vi "PCO_SetADCOperation.vi"(8 "error in (no error)":errorcluster {"code" format="%x"}, 10 "wADCOperation":u16(ring) items=["", "single ADC", "dual ADC"], 11 "ph":u64) -> (0 "error out":errorcluster {"code" format="%x"}, 2 "ErrorMessage":i32 format="%x", 3 "ph out":u64)   [LabVIEW 2019, in "SDK.lvlib" / "ImageSensor.lvlib"]
doc: "<b>Description:</b>\nThis function does set the ADC (analog-digital-converter) operating mode. Possible values are given through the parameter wNumADCsDESC of the PCO_Description structure. If sensor data is read out using single ADC operation linearity of image data is enhanced, using dual ADC operation readout is faster and allows higher frame rates. If dual ADC operating mode is set, horizontal ROI must be adapted to symmetrical values.\n\n<b>Supported camera type:</b>\npco.1600, pco.2000, pco.4000\n\n<b>Descriptor dependency:</b>\nwNumADCsDESC"
uses:
  ImageSensor.lvlib
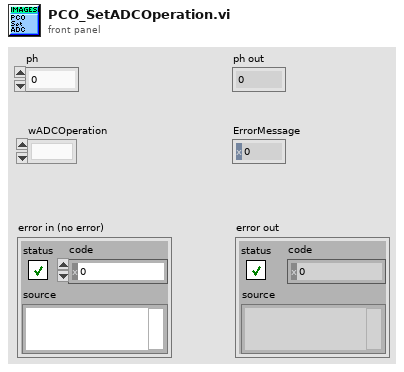
[diagram p1: front panel]
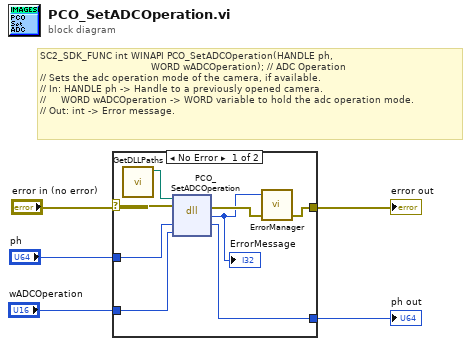
[diagram p0: block diagram]
diagram:
  # "SC2_SDK_FUNC int WINAPI PCO_SetADCOperation(HANDLE ph,\n                                     WORD wADCOperation); // ADC Operation\n// Sets the adc operation mode of the camera, if available.\n// In: HANDLE ph -> Handle to a previously opened camera.\n//     WORD wADCOperation -> WORD variable to hold the adc operation mode.\n// Out: int -> Error message."
  n1 = case shown="No Error" "error in (no error)" {
    selector: "error in (no error)" -> [w10 w15]
    tunnel: "ph" -> [w13 w14]
    tunnel: [w12 w14] -> w4
    tunnel: "wADCOperation" -> [w11 _]
    tunnel: [w8 w15] -> w2
    frame No Error {
      n2 = call "GetDLLPaths.vi"() -> ("SC2_Cam_Path"=w6:path)  [unwired: 9 in, 2 out]
      n3 = dll-call lib="?" fn="PCO_SetADCOperation"(path in=w6, error in=w10, "ph"=w13, "wADCOperation"=w11) -> (error out=w9:errorcluster, "return type"=w7:i32, "ph"=w12:u64)  [unwired: 2 in, 1 out]
      "ErrorMessage" <- w7
      n4 = call "ErrorManager.vi"("error in (no error)"=w9, "error code"=w7) -> ("error out"=w8:errorcluster)  [unwired: 3 in]
    }
    frame Error {
    }
  }
  "ph out" <- w4
  "error out" <- w2
